vi "Crab.vi"(10 "J1 Y":dbl format="%#_f", 11 "J1 X":dbl) -> (2 "Magnitude":dbl, 3 "Joystick Degree":dbl)   [LabVIEW 2011, in "Pivot Drive.lvlib"]
uses:
  Pivot Drive.lvlib
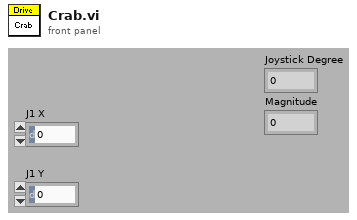
[diagram p1: front panel]
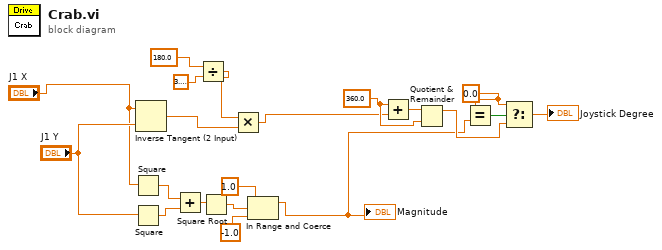
[diagram p0: block diagram]
diagram:
  w4 = 0.0
  w12 = 360.0
  n1 = Square(x="J1 X") -> (x^2=w15:dbl)
  n2 = Square(x="J1 Y") -> (x^2=w16:dbl)
  n3 = Inverse Tangent (2 Input)(1:"J1 Y", 2:"J1 X") -> (0:w17:dbl)
  n4 = Add(x=w15, y=w16) -> (x+y=w14:dbl)
  n5 = Divide(x=180.0, y=3.141592653589793) -> (x/y=w18:dbl)
  n6 = Square Root(x=w14) -> (sqrt(x)=w7:dbl)
  n7 = Multiply(x=w18, y=w17) -> (x*y=w11:dbl)
  n8 = In Range and Coerce(upper limit=1.0, x=w7, lower limit=-1.0 ("upper limit")) -> (coerced(x)=w3:dbl)  [unwired: 1 out]
  "Magnitude" <- w3
  n9 = Add(x=w12, y=w11) -> (x+y=w13:dbl)
  n10 = Quotient & Remainder(x=w13, y=w12) -> (x-y*floor(x/y)=w8:dbl)  [unwired: 1 out]
  n11 = Equal?(x=w4, y=w3) -> (x = y?=w10:bool)
  n12 = Select(t=w4, s=w10, f=w8) -> (s? t:f=→"Joystick Degree":dbl)
